vi "PD.vi"() -> ()   [LabVIEW 2019]
uses:
  <vilib>/Platform/TimedLoop/XDataNode/timing_clust.ctl
  <vilib>/Platform/TimedLoop/XDataNode/nitl_modes.ctl
  <vilib>/Platform/TimedLoop/XDataNode/wakeup.ctl
  <vilib>/myRIO/Instrument Drivers/Onboard IO/DIO/typedefs/DIO Reference.ctl
  <vilib>/myRIO/Common/Instrument Driver Framework/Utilities/typedefs/myRIO Generic Hardware Reference.ctl
  <vilib>/myRIO/Common/Instrument Driver Framework/Utilities/typedefs/Hardware Version Enum.ctl
  <vilib>/myRIO/Common/Instrument Driver Framework/Utilities/typedefs/myRIO v1.0 Reference.ctl
  <vilib>/myRIO/Common/Instrument Driver Framework/Utilities/typedefs/Generic FPGA Reference.ctl
  <vilib>/myRIO/Common/Instrument Driver Framework/myRIO v1.0/DIO/typedefs/DIO Channels List.ctl
  <vilib>/myRIO/Common/Instrument Driver Framework/myRIO v1.0/DIO/typedefs/DIO Channels Enum.ctl
  <vilib>/userDefined/High Color/nirio_resource_hc.ctl
  <vilib>/myRIO/Instrument Drivers/Onboard IO/AI/typedefs/AI Reference.ctl
  <vilib>/myRIO/Common/Instrument Driver Framework/myRIO v1.0/AI/typedefs/AI Channels List.ctl
  <vilib>/myRIO/Common/Instrument Driver Framework/myRIO v1.0/AI/typedefs/AI Channels Enum.ctl
  <vilib>/myRIO/Common/Instrument Driver Framework/Utilities/typedefs/Analog Scaling Constants List.ctl
  <vilib>/myRIO/Common/Instrument Driver Framework/Utilities/typedefs/Analog Scaling Constants.ctl
  <vilib>/Simulation/Shared/_Datatypes/SIM SISO Transfer Function.ctl
  <vilib>/myRIO/Instrument Drivers/Onboard IO/AO/typedefs/AO Reference.ctl
  <vilib>/myRIO/Common/Instrument Driver Framework/myRIO v1.0/AO/typedefs/AO Channels List.ctl
  <vilib>/myRIO/Common/Instrument Driver Framework/myRIO v1.0/AO/typedefs/AO Channels Enum.ctl
  <vilib>/myRIO/Common/Instrument Driver Framework/Utilities/vis/Is FPGA Ref Available.vi
  <vilib>/myRIO/Common/Instrument Driver Framework/myRIO v1.0/AI/vis/myRIO v1.1 Open AI.vi
  <vilib>/myRIO/Instrument Drivers/Onboard IO/AI/vis/Read.vi
  <vilib>/myRIO/Common/Instrument Driver Framework/myRIO v1.0/DIO/vis/myRIO v1.1 Open DIO.vi
  <vilib>/myRIO/Instrument Drivers/Onboard IO/DIO/vis/Write.vi
  <vilib>/Simulation/DiscreteLinear/Implementation/NILVSim Discrete Transfer Function Direct.llb/SIM Discrete Transfer Function Diagram (SISO).vi
  <vilib>/myRIO/Common/Instrument Driver Framework/myRIO v1.0/AO/vis/myRIO v1.1 Open AO.vi
  <vilib>/myRIO/Instrument Drivers/Onboard IO/AO/vis/Write.vi
  <vilib>/myRIO/Common/Instrument Driver Framework/Utilities/vis/Validate Channels.vi
  <vilib>/myRIO/Common/Instrument Driver Framework/myRIO v1.0/AI/vis/myRIO v1.0 Reserve AI.vi
  <vilib>/myRIO/Common/Instrument Driver Framework/myRIO v1.0/DIO/vis/myRIO v1.0 Reserve DIO.vi
  <vilib>/Simulation/ContinuousLinear/Implementation/Shared/SIM Transfer Function Support.llb/SIM TransferFunction Normalize to Buffer.vi
  <vilib>/Simulation/DiscreteLinear/Implementation/Shared/SIM Init Discrete States.vi
  <vilib>/Simulation/DiscreteLinear/Implementation/NILVSim Discrete Transfer Function Direct.llb/SIM Transfer Function Direct core (SISO).vi
  <vilib>/myRIO/Common/Instrument Driver Framework/myRIO v1.0/AO/vis/myRIO v1.0 Reserve AO.vi
  <vilib>/myRIO/Common/Instrument Driver Framework/myRIO v1.0/AI/vis/myRIO v1.0 Build MUX Configuration AI.vi
  <vilib>/myRIO/Common/Instrument Driver Framework/myRIO v1.0/Resource Manager/vis/myRIO v1.0 Reserve Channel List.vi
  <vilib>/myRIO/Common/Instrument Driver Framework/myRIO v1.0/DIO/vis/myRIO v1.0 Build MUX Configuration DIO.vi
  <vilib>/Simulation/ContinuousLinear/Implementation/Shared/SIM Transfer Function Support.llb/SIM TransferFunction Normalize.vi
  <vilib>/myRIO/Common/Instrument Driver Framework/myRIO v1.0/AO/vis/myRIO v1.0 Build MUX Configuration AO.vi
  <vilib>/myRIO/Common/Instrument Driver Framework/myRIO v1.0/Resource Manager/vis/myRIO v1.0 Reserve Channel.vi
  <vilib>/myRIO/Common/Instrument Driver Framework/myRIO v1.0/Resource Manager/vis/myRIO v1.0 Unreserve Channel.vi
  <vilib>/myRIO/Common/Instrument Driver Framework/myRIO v1.0/Resource Manager/vis/myRIO v1.0 Create Configuration List.vi
  <vilib>/Simulation/Implementation/Shared/SIM Polynomials.llb/SIM Remove Zero Coefficients (DBL).vi
  <vilib>/myRIO/Common/Instrument Driver Framework/myRIO v1.0/Resource Manager/vis/myRIO v1.0 Build Mutex Name.vi
  <vilib>/Utility/VariantDataType/GetNumericInfo.vi
  <vilib>/Utility/error.llb/Error Cluster From Error Code.vi
  <vilib>/myRIO/Common/Instrument Driver Framework/myRIO v1.0/myRIO v1.1 Open.vi
  <vilib>/myRIO/Common/Instrument Driver Framework/Utilities/vis/IO Manager.vi
  <vilib>/myRIO/Common/Instrument Driver Framework/Utilities/vis/Configuration Manager.vi
  <vilib>/myRIO/Common/Instrument Driver Framework/myRIO v1.0/Resource Manager/vis/myRIO v1.0 Configure IO.vi
  <vilib>/myRIO/Common/Instrument Driver Framework/myRIO v1.0/myRIO v1.0 Close.vi
  <vilib>/myRIO/Common/Instrument Driver Framework/myRIO v1.0/DIO/vis/myRIO v1.0 Write DIO.vi
  <vilib>/myRIO/Common/Instrument Driver Framework/myRIO v1.0/AI/vis/myRIO v1.0 Get Scaling Constants AI.vi
  <vilib>/myRIO/Common/Instrument Driver Framework/myRIO v1.0/AI/vis/myRIO v1.0 Read AI.vi
  <vilib>/Simulation/Implementation/Shared/SIM Polynomials.llb/SIM Divide Polynomials (DBL).vi
  <vilib>/Simulation/Implementation/Shared/SIM BuildSimErr.vi
  <vilib>/myRIO/Common/Instrument Driver Framework/myRIO v1.0/AO/vis/myRIO v1.0 Get Scaling Constants AO.vi
  <vilib>/myRIO/Common/Instrument Driver Framework/myRIO v1.0/AO/vis/myRIO v1.0 Write AO.vi
  <vilib>/platform/TimedLoop/XDataNode/XDataNode.xnode
  <vilib>/myRIO/Express VI/Onboard Devices/LED/LED Express VI.xnode
  <vilib>/myRIO/Instrument Drivers/Onboard IO/DIO/vis/myRIO DIO Open.xnode
  <vilib>/myRIO/Express VI/Onboard IO/AI/AI Express VI.xnode
  <vilib>/myRIO/Instrument Drivers/Onboard IO/AI/vis/myRIO AI Open.xnode
  <vilib>/Simulation/Implementation/XNodeFramework/SimXNode/SimX.xnode
  <vilib>/myRIO/Express VI/Onboard IO/AO/AO Express VI.xnode
  <vilib>/myRIO/Instrument Drivers/Onboard IO/AO/vis/myRIO AO Open.xnode
  <vilib>/Platform/TimedLoop/XDataNode/XDNodeRunTimeDep.lvlib
  <vilib>/myRIO/Instrument Drivers/Onboard IO/AI/AI.lvlib
  <vilib>/myRIO/Instrument Drivers/Onboard IO/AO/AO.lvlib
  <vilib>/myRIO/Instrument Drivers/Onboard IO/DIO/DIO.lvlib
panel:
  in  "LED0":bool
  in  "y":u32
  in  "Stop ADD":bool
  out "Current Output ADD":dbl(graph)=-0.0
  in  "Max FRF current 0-1000mA":dbl=10.0
  in  "Stop FRF":bool
  in  "esc":bool
  out "x[um]":dbl(graph)=2.4390249999999867
  out "Current Output EM":dbl(graph)=-0.0
  in  "Stop EM + FRF":bool=TRUE
  out "left[V]":dbl=-0.00025
  out "right[V]":dbl=-0.00025
  in  "initialize z":bool
  out "um":dbl=366.210975
  # "mA"
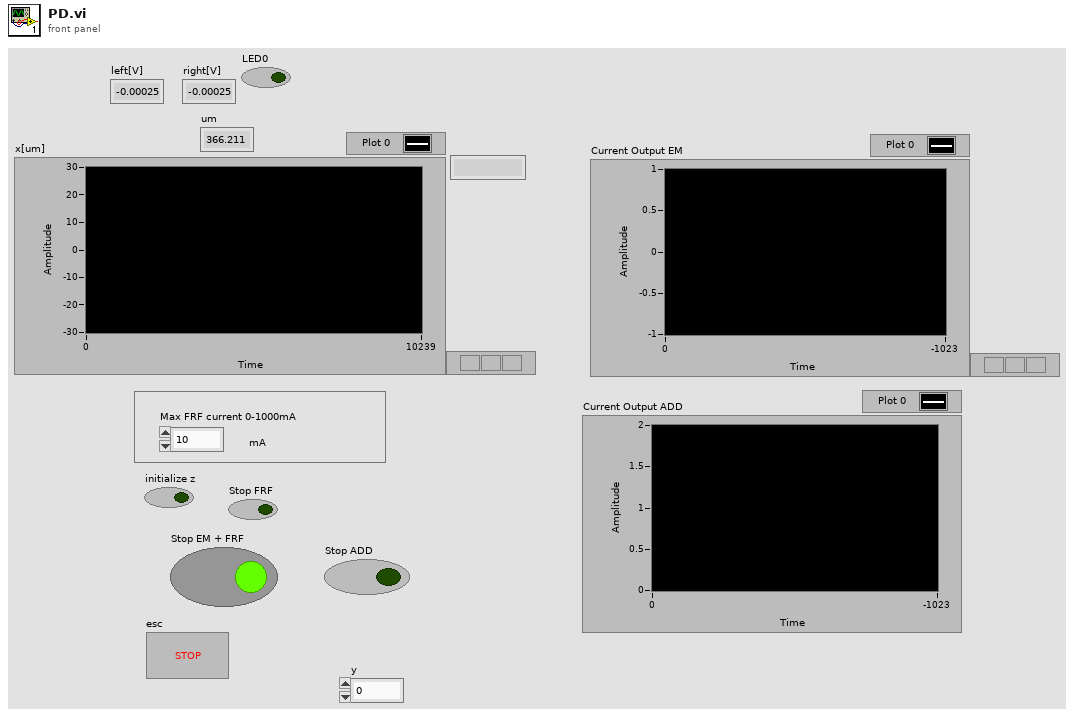
[diagram p1: front panel]
types:
  T1 = typedef "XDNodeRunTimeDep.lvlib/timing_clust.ctl" = cluster{"Expected End [f-1]":u64, "Actual End [f-1]":u64, "Finished Late? [f-1]":bool, "Expected End [i-1]":u64, "Actual End [i-1]":u64, "Finished Late? [i-1]":bool, "Expected Start [i]":u64, "Actual Start [i]":u64, "Expected Start [f]":u64, "Actual Start [f]":u64, "Source Name":string, "Structure Name":string, "Period":i64, "Deadline":i64, "Offset":i64, "Start":i64, "Priority":i32, "Timeout":i32, "Mode":T2, "Wakeup Reason":T3, "Error":errorcluster, "Source Type":string, "Secondary Source Type":string, "Global End Time":u64, "Global Start Time":u64, "Frame Duration":u64, "Iteration Duration":u64, "Assigned CPU":i32, "I/O Scan Engine Mode":u32}
  T2 = typedef "XDNodeRunTimeDep.lvlib/nitl_modes.ctl" = enum32{"No Change", "Process missed periods, maintain original phase", "Discard missed periods, maintain original phase", "Process missed periods, ignore original phase", "Discard missed periods, ignore original phase"}
  T3 = typedef "XDNodeRunTimeDep.lvlib/wakeup.ctl" = enum32{"Normal", "Aborted", "Asynchronous wakeup", "Timing source error", "Timed loop error", "Timeout"}
  T4 = typedef "DIO.lvlib/DIO Reference.ctl" = cluster{"myRIO Reference":T5, "DIO Channels List":T9}
  T5 = typedef "myRIO Generic Hardware Reference.ctl" = cluster{"myRIO Model":T6, "myRIO Hardware Reference":T7}
  T6 = typedef "Hardware Version Enum.ctl" = enum16{"Unknown", "myRIO-1900", "myRIO-1950", "roboRIO", "NI ELVIS RIO CM", "ELVIS III"}
  T7 = typedef "myRIO v1.0 Reference.ctl" = cluster{"Generic FPGA Reference":T8, "Allow multiple opens":bool}
  T8 = typedef "Generic FPGA Reference.ctl" = refnum<k20>
  T9 = typedef "DIO Channels List.ctl" = T10[]
  T10 = typedef "DIO Channels Enum.ctl" = enum16{"Not Connected", "C/DIO0", "C/DIO1", "C/DIO2", "C/DIO3", "C/DIO4", "C/DIO5", "C/DIO6", "C/DIO7", "A/DIO0", "A/DIO1", "A/DIO2", "A/DIO3", "A/DIO4", "A/DIO5", "A/DIO6", "A/DIO7", "A/DIO8", "A/DIO9", "A/DIO10", "A/DIO11", "A/DIO12", "A/DIO13", "A/DIO14", "A/DIO15", "A/DIO16", "A/DIO17", "A/DIO18", "A/DIO19", "B/DIO0", "B/DIO1", "B/DIO2", "B/DIO3", "B/DIO4", "B/DIO5", "B/DIO6", "B/DIO7", "B/DIO8", "B/DIO9", "B/DIO10", "B/DIO11", "B/DIO12", "B/DIO13", "B/DIO14", "B/DIO15", "B/DIO16", "B/DIO17", "B/DIO18", "B/DIO19", "LED0", "LED1", "LED2", "LED3", "Button0", "DIO/DIO0", "DIO/DIO1", "DIO/DIO2", "DIO/DIO3", "DIO/DIO4", "DIO/DIO5", "DIO/DIO6", "DIO/DIO7", "DIO/DIO8", "DIO/DIO9", "SPI/CS0", "SPI/CS1", "SPI/CS2", "SPI/CS3", "LED RADIO (Green)", "LED RADIO (Red)", "LED COMM (Green)", "LED COMM (Red)", "LED MODE (Green)", "LED MODE (Red)"}
  T11 = typedef "nirio_resource_hc.ctl" = tag
  T12 = typedef "SIM SISO Transfer Function.ctl" = cluster{"Numerator":dbl[], "Denominator":dbl[]}
  T13 = typedef "AO.lvlib/AO Reference.ctl" = cluster{"myRIO Reference":T5, "AO Channel List":T14, "AO Scaling Constant List":T16}
  T14 = typedef "AO Channels List.ctl" = T15[]
  T15 = typedef "AO Channels Enum.ctl" = enum16{"Not Connected", "AudioOut/Left", "AudioOut/Right", "C/AO0", "C/AO1", "A/AO0", "A/AO1", "B/AO0", "B/AO1"}
  T16 = typedef "Analog Scaling Constants List.ctl" = T17[]
  T17 = typedef "Analog Scaling Constants.ctl" = cluster{"LSB Weight (Volts)":dbl, "Offset (Volts)":dbl, "Signed?":bool}
  T18 = typedef "AI.lvlib/AI Reference.ctl" = cluster{"myRIO Reference":T5, "AI Channels List":T19, "AI Scaling Constants List":T16}
  T19 = typedef "AI Channels List.ctl" = T20[]
  T20 = typedef "AI Channels Enum.ctl" = enum16{"Not Connected", "AudioIn/Left", "AudioIn/Right", "C/AI0", "C/AI1", "A/AI0", "A/AI1", "A/AI2", "A/AI3", "A/AI4", "A/AI5", "A/AI6", "A/AI7", "B/AI0", "B/AI1", "B/AI2", "B/AI3", "B/AI4", "B/AI5", "B/AI6", "B/AI7", "AI/AI0", "AI/AI1", "AI/AI2", "AI/AI3", "A/AI0 (DIFF)", "A/AI1 (DIFF)", "A/AI2 (DIFF)", "A/AI3 (DIFF)", "B/AI0 (DIFF)", "B/AI1 (DIFF)", "B/AI2 (DIFF)", "B/AI3 (DIFF)"}
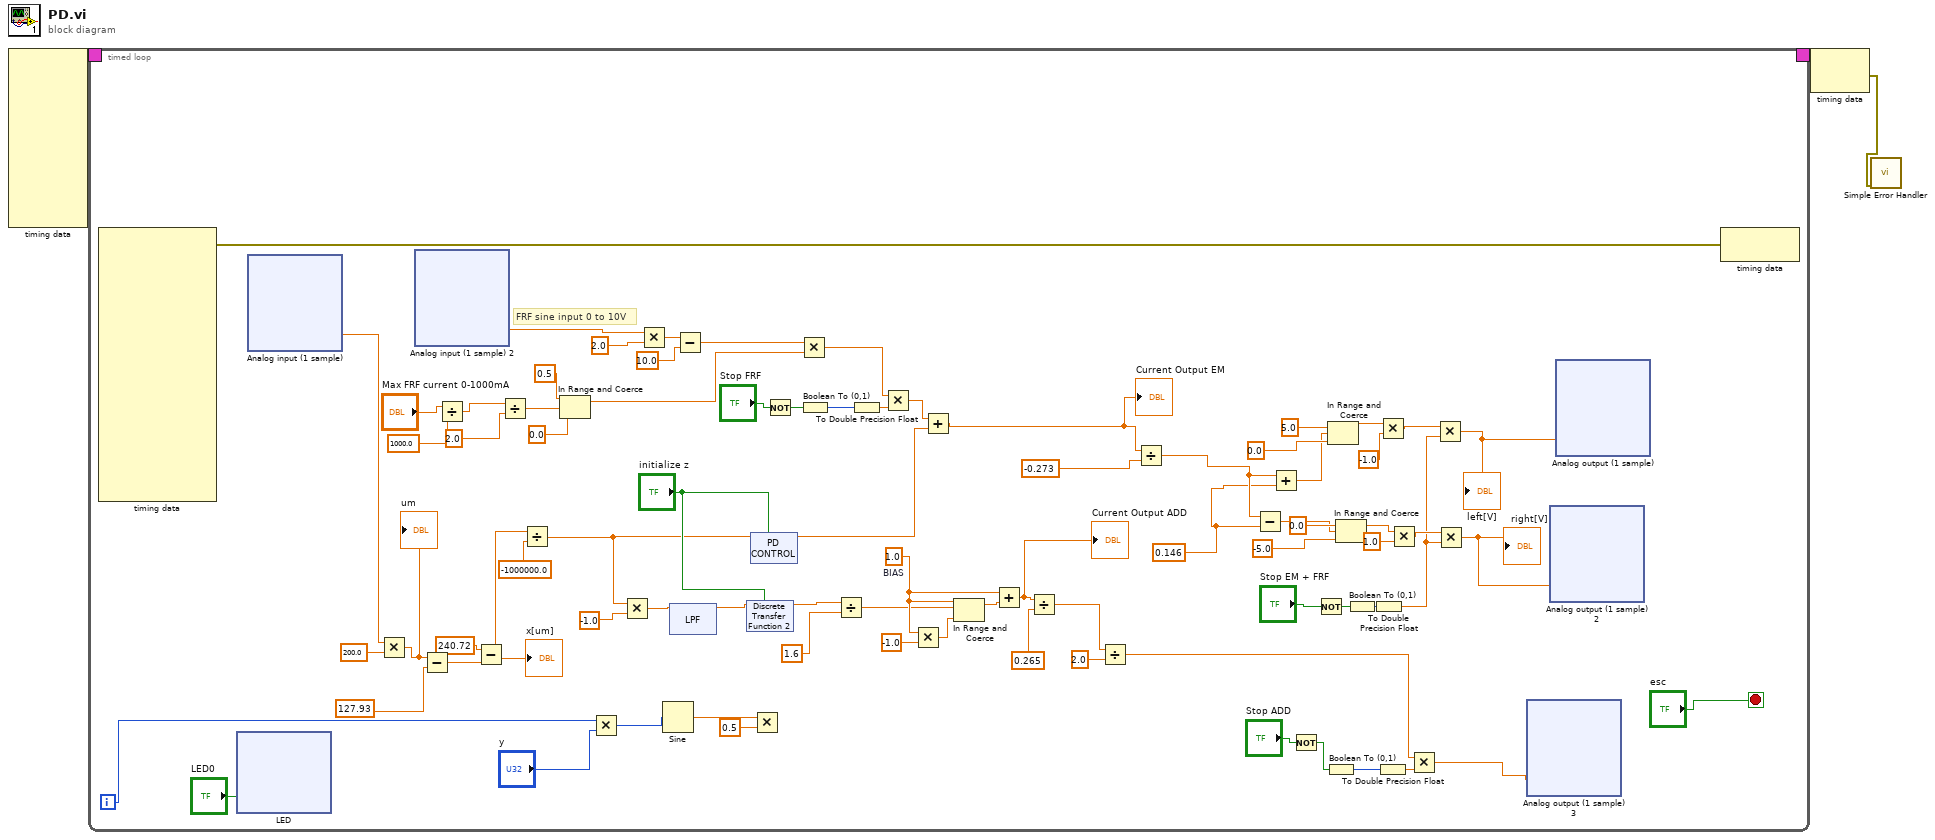
[diagram p0: block diagram]
diagram:
  n1 = node-c288() -> (w3:T1)  [unwired: 10 in]
  n2 = timed-loop {
    timing: w3 -> [_]
    timing-out: [_] -> w2
    i -> [w11]
    stop <- "esc" stop-if-true
    w26 = 1.0  # BIAS
    w41 = 0.146 ("y")
    # "FRF sine input 0 to 10V"
    n3 = node-c288() -> (w83:errorcluster)  [unwired: 1 in, 16 out]
    n4 = xnode "LED"("LED0"="LED0") -> ()  [unwired: 1 in, 1 out]
    n5 = xnode "Analog input (1 sample)"() -> ("C/AI1 (AI1)"=w36:dbl)  [unwired: 1 in, 1 out]
    n6 = Multiply(x=w36, y=200.0) -> (x*y=w81:dbl)
    "um" <- w81
    n7 = xnode "Analog input (1 sample) 2"() -> ("C/AI0 (AI0)"=w60:dbl)  [unwired: 1 in, 1 out]
    n8 = Subtract(x=w81, y=127.93) -> (x-y=w80:dbl)
    n9 = Divide(x="Max FRF current 0-1000mA", y=1000.0) -> (x/y=w49:dbl)
    n10 = Subtract(x=240.72, y=w80) -> (x-y=w35:dbl)
    "x[um]" <- w35
    n11 = Divide(x=w49, y=2.0) -> (x/y=w53:dbl)
    n12 = Divide(x=w35, y=-1000000.0) -> (x/y=w33:dbl)
    n13 = In Range and Coerce(upper limit=0.5, x=w53, lower limit=0.0) -> (coerced(x)=w50:dbl)  [unwired: 1 out]
    n14 = Multiply(x=w11, y="y") -> (x*y=w13:u32)
    n15 = Multiply(x=w33, y=-1.0) -> (x*y=w17:dbl)
    n16 = Multiply(x=w60, y=2.0) -> (x*y=w58:dbl)
    n17 = Sine(x=w13) -> (sin(x)=w15:dbl)
    n18 = xnode "LPF"("input u(k)"=w17) -> ("output y(k)"=w16:dbl)  [unwired: 2 in, 1 out]
    n19 = Subtract(x=w58, y=10.0) -> (x-y=w55:dbl)
    n20 = xnode ("Discrete Transfer Function 2")("input u(k)"=w16, "initialize"="initialize z") -> ("output y(k)"=w32:dbl)  [unwired: 1 in, 1 out]
    n21 = xnode "PD CONTROL"("input u(k)"=w33, "initialize"="initialize z") -> ("output y(k)"=w42:dbl)  [unwired: 1 in, 1 out]
    n22 = Multiply(x=w15, y=0.5) -> ()  [unwired: 1 out]
    n23 = Not(x="Stop FRF") -> (.not. x?=w63:bool)
    n24 = Multiply(x=w55, y=w50) -> (x*y=w56:dbl)
    n25 = Boolean To (0,1)(Boolean=w63) -> (0, 1=w62:i16)
    n26 = Divide(x=w32, y=1.6) -> (x/y=w10:dbl)
    n27 = To Double Precision Float(number=w62) -> (double precision float=w61:dbl)
    n28 = Multiply(x=w56, y=w61) -> (x*y=w65:dbl)
    n29 = Multiply(x=w26, y=-1.0) -> (x*y=w27:dbl)
    n30 = Add(x=w65, y=w42) -> (x+y=w40:dbl)
    "Current Output EM" <- w40
    n31 = In Range and Coerce(upper limit=w26, x=w10, lower limit=w27) -> (coerced(x)=w29:dbl)  [unwired: 1 out]
    n32 = Add(x=w26, y=w29) -> (x+y=w28:dbl)
    "Current Output ADD" <- w28
    n33 = Divide(x=w28, y=0.265) -> (x/y=w9:dbl)
    n34 = Divide(x=w9, y=2.0) -> (x/y=w8:dbl)
    n35 = Divide(x=w40, y=-0.273) -> (x/y=w43:dbl)
    n36 = Subtract(x=w43, y=w41) -> (x-y=w44:dbl)
    n37 = Add(x=w43, y=w41) -> (x+y=w45:dbl)
    n38 = Not(x="Stop ADD") -> (.not. x?=w22:bool)
    n39 = Not(x="Stop EM + FRF") -> (.not. x?=w68:bool)
    n40 = Boolean To (0,1)(Boolean=w22) -> (0, 1=w21:i16)
    n41 = In Range and Coerce(upper limit=5.0 ("x"), x=w45, lower limit=0.0) -> (coerced(x)=w5:dbl)  [unwired: 1 out]
    n42 = In Range and Coerce(upper limit=0.0 ("x"), x=w44, lower limit=-5.0) -> (coerced(x)=w73:dbl)  [unwired: 1 out]
    n43 = Boolean To (0,1)(Boolean=w68) -> (0, 1=w70:i16)
    n44 = To Double Precision Float(number=w70) -> (double precision float=w37:dbl)
    n45 = Multiply(x=w5, y=-1.0) -> (x*y=w39:dbl)
    n46 = To Double Precision Float(number=w21) -> (double precision float=w20:dbl)
    n47 = Multiply(x=w73, y=1.0) -> (x*y=w38:dbl)
    n48 = Multiply(x=w8, y=w20) -> (x*y=w6:dbl)
    n49 = Multiply(x=w39, y=w37) -> (x*y=w19:dbl)
    "left[V]" <- w19
    n50 = Multiply(x=w38, y=w37) -> (x*y=w18:dbl)
    "right[V]" <- w18
    n51 = xnode "Analog output (1 sample) 3"("A/AO1 (Pin 4)"=w6) -> ()  [unwired: 1 in, 1 out]
    n52 = xnode "Analog output (1 sample) 2"("C/AO1 (AO1)"=w18) -> ()  [unwired: 1 in, 1 out]
    n53 = xnode "Analog output (1 sample)"("C/AO0 (AO0)"=w19) -> ()  [unwired: 1 in, 1 out]
    n54 = node-c288(w83) -> ()  [unwired: 1 out]
  }
  n55 = node-c288(w2) -> (w1:errorcluster)
  n56 = call <vilib>:"Simple Error Handler.vi"("error in (no error)"=w1) -> ()  [unwired: 4 in, 5 out]
